vi "Move and Rename Text File.vi"(7 "Project Name":string="123", 8 "error in (no error)":errorcluster, 10 "Project":refnum<vi>, 11 "Template INI Path":path=path "C:/LabView data/EMD sub-base/123.txt") -> (0 "error out":errorcluster)   [LabVIEW 2020]
doc: "This VI will do the remove the ini file from Project, Rename the ini file with Project name after that again add the ini file into project."
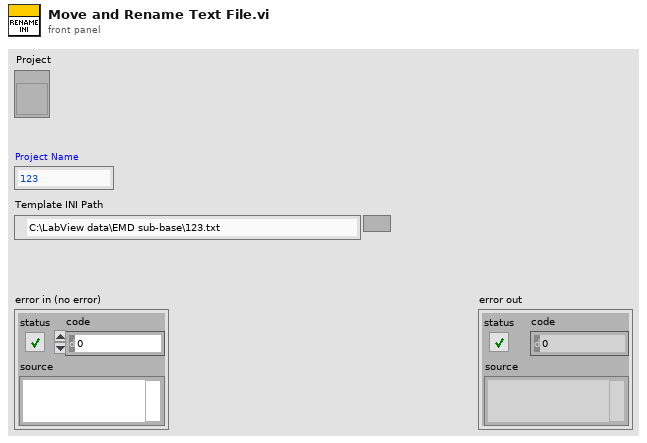
[diagram p1: front panel]
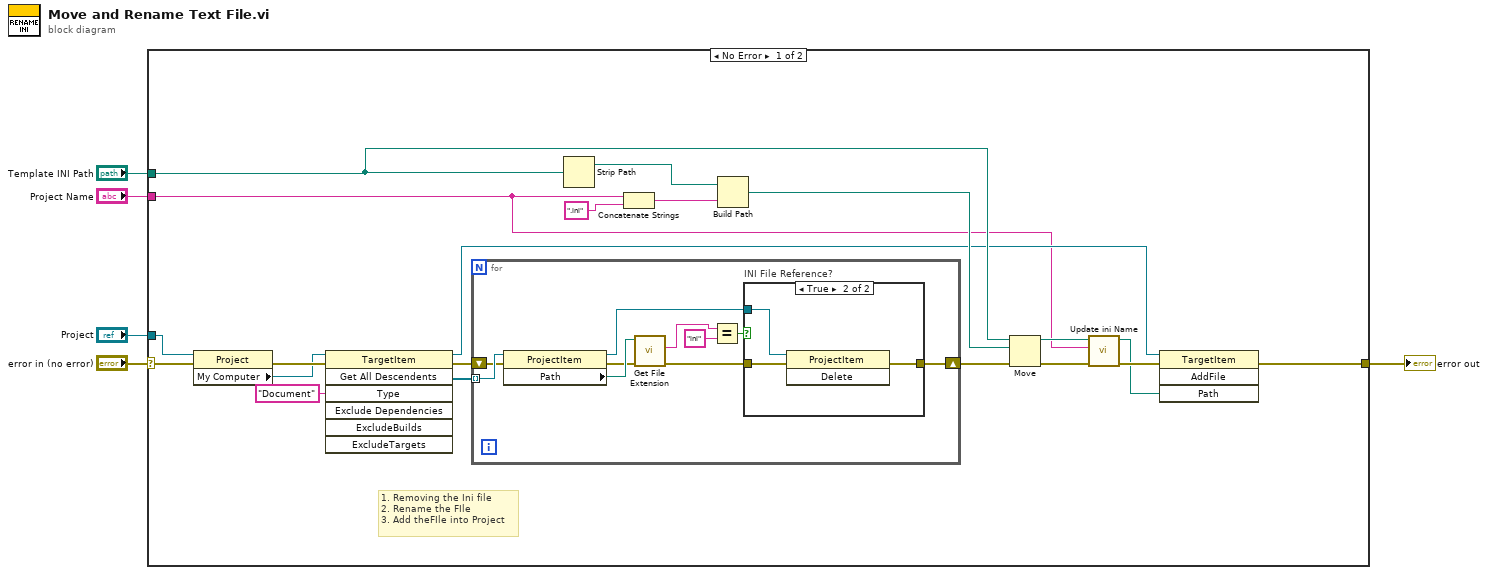
[diagram p0: block diagram]
diagram:
  n1 = case shown="No Error" "error in (no error)" {
    selector: "error in (no error)" -> [w18 w40]
    tunnel: "Project Name" -> [w6 _]
    tunnel: "Template INI Path" -> [w22 _]
    tunnel: [w12 w40] -> w2
    tunnel: "Project" -> [w13 _]
    frame No Error {
      # "1. Removing the Ini file \n2. Rename the FIle \n3. Add theFIle into Project"
      n2 = property class="Project"(reference=w13, error in=w18) -> (error out=w17:errorcluster, "My Computer"=w11:refnum<vi>)  [unwired: 1 out]
      n3 = invoke class="TargetItem" method="Get All Descendents"(reference=w11, error in=w17, "Type"="Document") -> (reference out=w14:refnum<vi>, error out=w16:errorcluster, "All Descendents"=w20:refnum<vi>[])  [unwired: 4 in, 4 out]
      n4 = for {
        tunnel: w20 -> [w35] mode=indexing
        shift-right: [w26] -> w15
        shift-left: w16 -> [w29]
        n5 = property class="ProjectItem"(reference=w35, error in=w29) -> (reference out=w30:refnum<vi>, error out=w28:errorcluster, "Path"=w31:path)
        n6 = call <vilib>:"Get File Extension.vi"("error in (no error)"=w28, "file"=w31) -> ("error out"=w27:errorcluster, "lowercase file extension"=w34:string)  [unwired: 5 in, 3 out]
        n7 = Equal?(x=w34, y="ini") -> (x = y?=w32:bool)
        n8 = case "INI File Reference?" shown="True" w32 {
          tunnel: w30 -> [_ w39]
          tunnel: w27 -> [w36 w38]
          tunnel: [w36 w37] -> w26
          frame False {
          }
          frame True {
            n9 = invoke class="ProjectItem" method="Delete"(reference=w39, error in=w38) -> (error out=w37:errorcluster)  [unwired: 1 in, 2 out]
          }
        }
      }
      n10 = Strip Path(path=w22) -> (stripped path=w23:path)  [unwired: 1 out]
      n11 = Concatenate Strings(w6, ".ini" ("string")) -> (w25:string)
      n12 = Build Path(base path=w23, name or relative path=w25) -> (appended path=w21:path)
      n13 = Move(source path=w22, error in=w15, 10:w21) -> (error out=w10:errorcluster, 3:w8:path)  [unwired: 2 in, 1 out]
      n14 = call "Update ini Name.vi"("error in (no error)"=w10, "Plugin Name"=w6, "configuration file path"=w8) -> ("error out"=w9:errorcluster, "configuration file path Out"=w7:path)  [unwired: 7 in]
      n15 = invoke class="TargetItem" method="AddFile"(reference=w14, error in=w9, "Path"=w7) -> (error out=w12:errorcluster)  [unwired: 1 in, 3 out]
    }
    frame Error {
    }
  }
  "error out" <- w2
